vi "Return_Data.vi"(8 "error in (no error)":errorcluster caption="entrée d'erreur (pas d'erreur)", 11 "Class Instrument Firebase Altyor en entrée":refnum<class "Class Instrument Firebase Altyor.lvclass">) -> (0 "error out":errorcluster caption="sortie d'erreur", 2 "Data_Json":string, 3 "Class Instrument Firebase Altyor en sortie":refnum<class "Class Instrument Firebase Altyor.lvclass">)   [LabVIEW 2020, in "Library Instrument & Equipement.lvlib" / "Library Instruments.lvlib" / "Class Instrument Firebase Altyor.lvclass"]
uses:
  Class Instrument Firebase Altyor.lvclass
  Class Instrument Firebase Altyor.lvclass/Class Instrument Firebase Altyor.ctl
  JSON API/Variant JSON/Variant to JSON.vi
  JSON API/JSON Value/Get Item by name array.vi
  Firebase/Source/Firebase Altyor/Firebase Altyor.lvclass
  JSON API/JSON Value/JSON Value.lvclass
  JSON API/Get Polymorphic/JSON GetSet.lvlib
  JSON API/Variant JSON/Variant JSON.lvlib
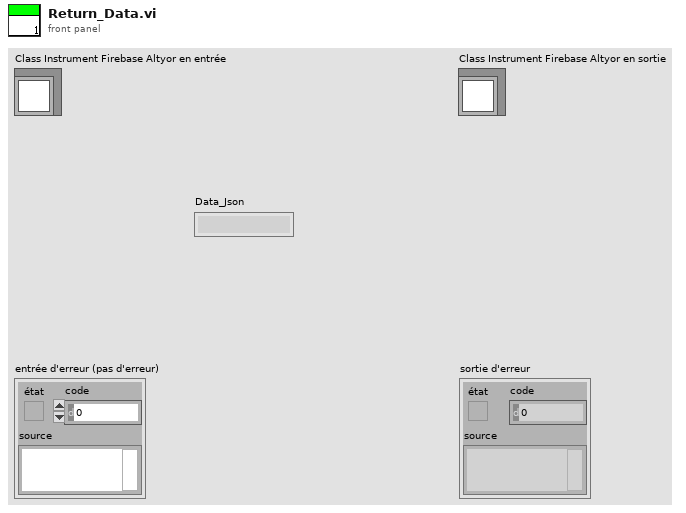
[diagram p1: front panel]
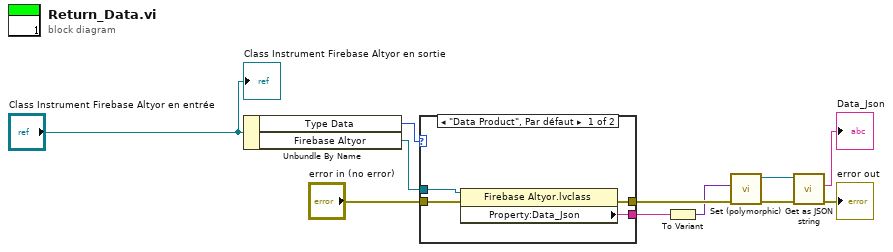
[diagram p0: block diagram]
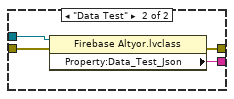
[diagram p2: hidden frame]
diagram:
  n1 = Unbundle By Name("Class Instrument Firebase Altyor en entrée") -> ("Type Data"=w11:enum16{"Data Product", "Data Test"}, "Firebase Altyor"=w9:refnum<class "Firebase Altyor.lvclass">)
  n2 = case shown="\"Data Product\", Par défaut" w11 {
    tunnel: w9 -> [w14 w19]
    tunnel: "error in (no error)" -> [w15 w18]
    tunnel: [w12 w17] -> w5
    tunnel: [w13 w16] -> w4
    frame "Data Product", Default {
      n3 = property class="Firebase Altyor.lvclass"(reference=w14, error in=w15) -> (error out=w12:errorcluster, "Property:Data_Json"=w13:string)  [unwired: 1 out]
    }
    frame "Data Test" {
      n4 = property class="Firebase Altyor.lvclass"(reference=w19, error in=w18) -> (error out=w17:errorcluster, "Property:Data_Test_Json"=w16:string)  [unwired: 1 out]
    }
  }
  n5 = To Variant(anything=w4) -> (Variant=w1:variant)
  n6 = call-poly "Set (polymorphic).vi"("error in (no error)"=w5, "Variant"=w1) -> ("error out"=w6:errorcluster, "JSON Value out"=w7:refnum<class "JSON Value.lvclass">)  [unwired: 8 in]
  n7 = call "Get as JSON string.vi"("error in (no error)"=w6, "JSON Value in"=w7) -> ("error out"=→"error out":errorcluster, "<JSON>"=→"Data_Json":string)  [unwired: 8 in]
  "Class Instrument Firebase Altyor en sortie" <- "Class Instrument Firebase Altyor en entrée"
